vi "WiiMote Read Accelerometer Buttons and Balance.vi"(0 "Wiimote":refnum<k24>, 11 "error in":errorcluster) -> (4 "reference out":refnum<k24>, 6 "Wiimote State":T2, 8 "Balance Board State":T1, 15 "error out":errorcluster)   [LabVIEW 2015]
doc: "Get accel / button state from wiimote \nSam Shearman"
uses:
  WiiMote State.ctl
  C:/Users/gilled/Downloads/EmbeddedLab_v1.70_Courseware-Kobuki/EmbeddedLab_v1.70_Courseware/Courseware/src/LabVIEW/WiiMote/Dependencies/WiimoteLib.dll
  Dependencies/WiimoteLib.dll
panel:
  # "Establish a Bluetooth link with your Wiimote prior to executing this VI.\n\nRequires the Wiimote Managed Library WiimoteLib Ver 1.7\navailable from http://www.codeplex.com/WiimoteLib\nSam Shearman"
  # "Accelerometers"
  # "Buttons"
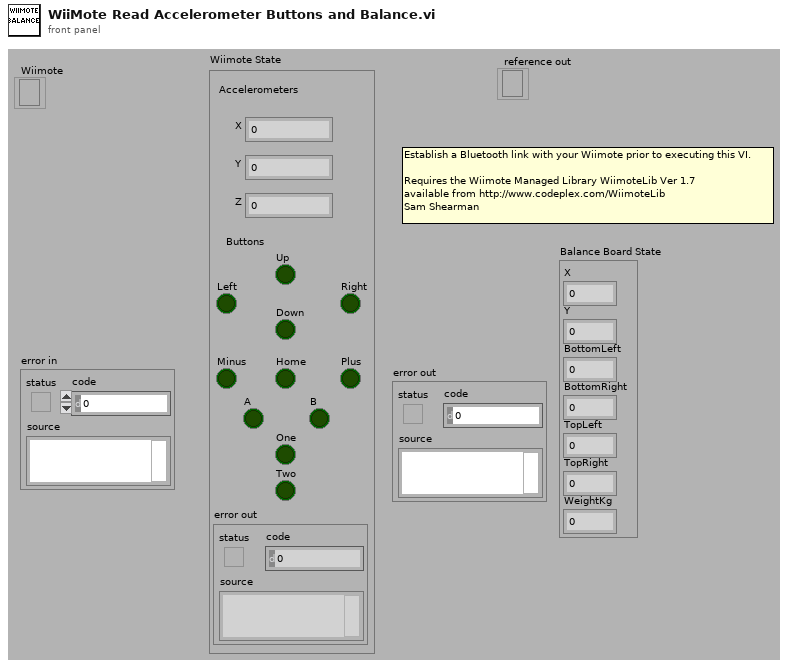
[diagram p1: front panel]
types:
  T1 = cluster{"X":sgl, "Y":sgl, "BottomLeft":sgl, "BottomRight":sgl, "TopLeft":sgl, "TopRight":sgl, "WeightKg":sgl}
  T2 = typedef "WiiMote State.ctl" = cluster{"X":sgl, "Y":sgl, "Z":sgl, "A":bool, "B":bool, "Down":bool, "Home":bool, "Left":bool, "Minus":bool, "One":bool, "Plus":bool, "Right":bool, "Two":bool, "Up":bool, "error out":errorcluster}
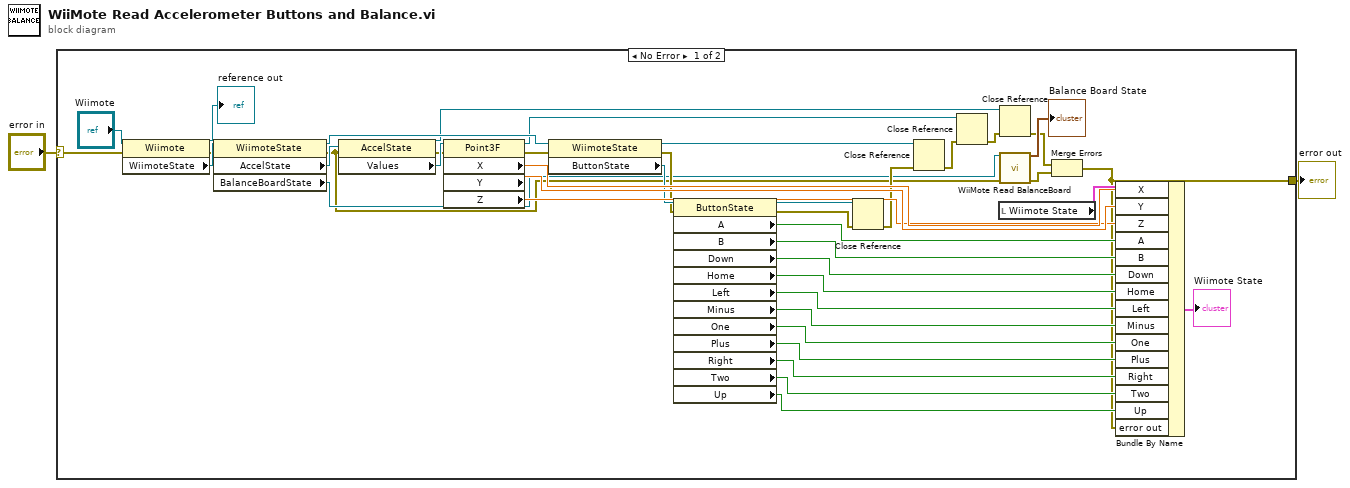
[diagram p0: block diagram]
diagram:
  n1 = case shown="No Error" "error in" {
    selector: "error in" -> [w12 w45]
    tunnel: [w3 w45] -> w2
    frame No Error {
      n2 = property class="Wiimote"(reference="Wiimote", error in=w12) -> (reference out=→"reference out":refnum<k24>, error out=w25:errorcluster, "WiimoteState"=w26:refnum<k24>)
      n3 = property class="WiimoteState"(reference=w26, error in=w25) -> (reference out=w23:refnum<k24>, error out=w7:errorcluster, "AccelState"=w31:refnum<k24>, "BalanceBoardState"=w8:refnum<k24>)
      n4 = property class="AccelState"(reference=w31, error in=w7) -> (reference out=w17:refnum<k24>, error out=w16:errorcluster, "Values"=w30:refnum<k24>)
      n5 = property class="Point3F"(reference=w30, error in=w16) -> (reference out=w14:refnum<k24>, error out=w15:errorcluster, "X"=w29:sgl, "Y"=w28:sgl, "Z"=w27:sgl)
      n6 = property class="WiimoteState"(reference=w23, error in=w15) -> (reference out=w18:refnum<k24>, error out=w21:errorcluster, "ButtonState"=w22:refnum<k24>)
      n7 = property class="ButtonState"(reference=w22, error in=w21) -> (reference out=w19:refnum<k24>, error out=w13:errorcluster, "A"=w42:bool, "B"=w41:bool, "Down"=w40:bool, "Home"=w39:bool, "Left"=w38:bool, "Minus"=w37:bool, "One"=w36:bool, "Plus"=w35:bool, "Right"=w34:bool, "Two"=w33:bool, "Up"=w32:bool)
      n8 = Close Reference(reference=w19, error in (no error)=w13) -> (error out=w11:errorcluster)
      n9 = Close Reference(reference=w18, error in (no error)=w11) -> (error out=w10:errorcluster)
      n10 = Close Reference(reference=w14, error in (no error)=w10) -> (error out=w9:errorcluster)
      n11 = local read "Wiimote State"() -> (w43:T2)
      n12 = Close Reference(reference=w17, error in (no error)=w9) -> (error out=w5:errorcluster)
      n13 = call "WiiMote Read BalanceBoard.vi"("BalanceBoardState"=w8, "error in"=w7) -> ("Balance Board State"=→"Balance Board State":T1, "error out"=w4:errorcluster)  [unwired: 12 out]
      n14 = Merge Errors(w5, w4) -> (w3:errorcluster)
      n15 = Bundle By Name(cluster=w43, "X"=w29, "Y"=w28, "Z"=w27, "A"=w42, "B"=w41, "Down"=w40, "Home"=w39, "Left"=w38, "Minus"=w37, "One"=w36, "Plus"=w35, "Right"=w34, "Two"=w33, "Up"=w32, "error out"=w3) -> (→"Wiimote State":T2)
    }
    frame Error {
    }
  }
  "error out" <- w2
